vi "Check Link for Char or Meas.vi"(5 "Link":T1) -> (2 "Char?":bool)   [LabVIEW 2011]
uses:
  Controls/ECUMC Item.ctl
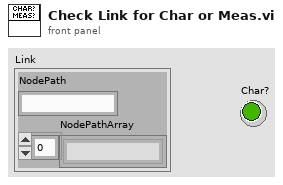
[diagram p1: front panel]
types:
  T1 = typedef "ECUMC Item.ctl" = cluster{"NodePath":string, "NodePathArray":string[]}
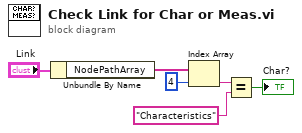
[diagram p0: block diagram]
diagram:
  n1 = Unbundle By Name("Link") -> ("NodePathArray"=w5:string[])
  n2 = Index Array(array=w5, index=4) -> (element=w3:string)
  n3 = Equal?(x=w3, y="Characteristics") -> (x = y?=→"Char?":bool)
